vi "nanomsg_sub_single.vi"() -> ()   [LabVIEW 2014]
uses:
  lvnanomsg/nanomsg_context.lvclass
  lvnanomsg/nanomsg_socket.lvclass
panel:
  out "data":string
  in  "port":i32=5555
  # "Nanomsg subscriber VI"
  # "Subscribe to all messages published to specified ports"
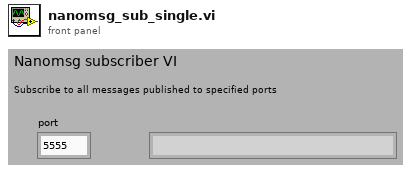
[diagram p1: front panel]
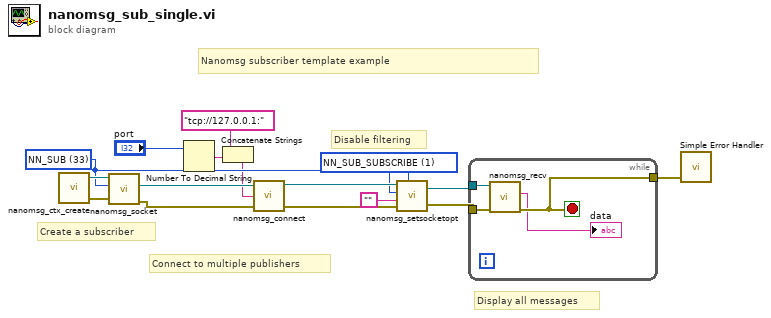
[diagram p0: block diagram]
diagram:
  w9 = 1 items=["NN_SUB_XXX", "NN_SUB_SUBSCRIBE", "NN_SUB_UNSUBSCRIBE"] ("option")
  w5 = 33 items=["NN_WS"=-4, "NN_TCP"=-3, "NN_IPC"=-2, "NN_INPROC"=-1, "NN_SOL_SOCKET"=0, "NN_PAIR"=16, "NN_PUB"=32, "NN_SUB"=33, "NN_REQ"=48, "NN_REP"=49, "NN_PUSH"=80, "NN_PULL"=81, "NN_SURVEYOR"=98, "NN_RESPONDENT"=99, "NN_BUS"=112] ("socket type")
  # "Nanomsg subscriber template example"
  # "Display all messages"
  # "Create a subscriber"
  # "Disable filtering"
  # "Connect to multiple publishers"
  n1 = call "nanomsg_ctx_create.vi"() -> ("error out"=w15:errorcluster, "context out"=w16:refnum<class "nanomsg_context.lvclass">)  [unwired: 4 in]
  n2 = call "nanomsg_socket.vi"("error in"=w15, "socket type"=w5, "context in"=w16) -> ("error out"=w14:errorcluster, "socket out"=w6:refnum<class "nanomsg_socket.lvclass">)  [unwired: 2 in, 1 out]
  n3 = Number To Decimal String(number="port") -> (decimal integer string=w2:string)  [unwired: 1 in]
  n4 = Concatenate Strings("tcp://127.0.0.1:" ("endpoint"), w2) -> (w3:string)
  n5 = call "nanomsg_connect.vi"("error in"=w14, "endpoint"=w3, "socket in"=w6) -> ("error out"=w12:errorcluster, "socket out"=w13:refnum<class "nanomsg_socket.lvclass">)  [unwired: 1 in]
  n6 = call "nanomsg_setsocketopt.vi"("socket in"=w13, "option"=w9, "value"="", "error in"=w12, "level"=w5) -> ("socket out"=w10:refnum<class "nanomsg_socket.lvclass">, "error out"=w11:errorcluster)
  n7 = while {
    tunnel: w10 -> [w20]
    tunnel: w11 -> [w19]
    tunnel: [w18] -> w7
    stop <- w18 stop-if-true
    n8 = call "nanomsg_recv.vi"("error in"=w19, "socket in"=w20) -> ("error out"=w18:errorcluster, "data"=→"data":string)  [unwired: 3 in, 3 out]
  }
  n9 = call <vilib>:"Simple Error Handler.vi"("error in (no error)"=w7) -> ()  [unwired: 4 in, 5 out]
